vi "instance count allowed.vi"(8 "error in":errorcluster, 11 "configuration in":refnum<class "PL_System Configuration.lvclass">) -> (0 "error out":errorcluster, 2 "instances allowed":i32, 3 "configuration out":refnum<class "PL_System Configuration.lvclass">)   [LabVIEW 2013, in "PL_System Configuration.lvclass"]
doc: "Provides an interface for determining the reentrancy of the runtime class associated with this configuration class. For example, a module which performs processing tasks may allow for unlimited instances (-1) while a component which implements a TCP server may want to limit itself to a smaller number in order to preserve ports. configuration.lvclass provides a value of 0, as no runtime class exists for this configuration."
uses:
  PL_System Configuration.lvclass
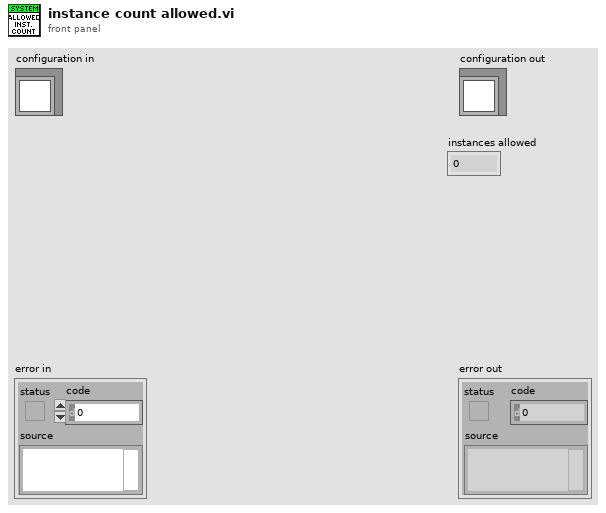
[diagram p1: front panel]
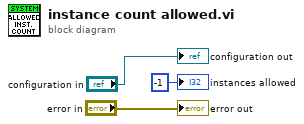
[diagram p0: block diagram]
diagram:
  "error out" <- "error in"
  "configuration out" <- "configuration in"
  "instances allowed" <- -1 ("instances allowed")
